vi "Get Active Project.vi"(11 "error in":errorcluster) -> (4 "name":string, 6 "path":path, 15 "error out":errorcluster)   [LabVIEW 2021, in "G-Plugin Editor.lvlib"]
uses:
  G-Plugin Editor.lvlib
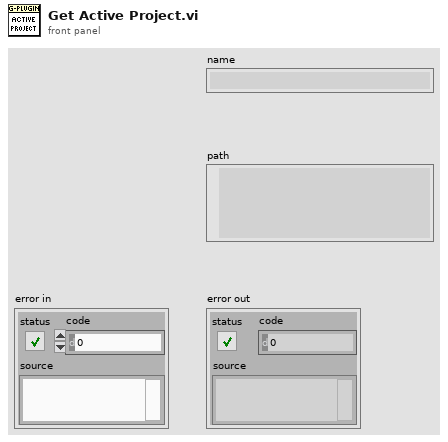
[diagram p1: front panel]
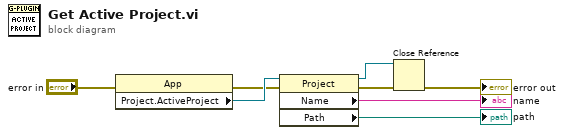
[diagram p0: block diagram]
diagram:
  n1 = property class="App"(error in="error in") -> (error out=w6:errorcluster, "Project.ActiveProject"=w7:refnum<vi>)  [unwired: 1 in, 1 out]
  n2 = property class="Project"(reference=w7, error in=w6) -> (reference out=w1:refnum<vi>, error out=w5:errorcluster, "Name"=→"name":string, "Path"=→"path":path)
  n3 = Close Reference(reference=w1, error in (no error)=w5) -> (error out=→"error out":errorcluster)
